vi "Self Fulfill Error.vi"(8 "error in (no error)":errorcluster) -> (0 "error out":errorcluster)   [LabVIEW 2017, in "Unit Tests.lvlib"]
uses:
  Unit Tests.lvlib
  e38c4525-3448-4fbc-8db8-7559fd649511.vi
  69632491-9656-44da-a05c-60cf6a618bb2.vi
  Promise Future/Promise/Promise.lvclass
  E:/Promise/Promise Future/Future/Future.lvclass
  Promise Future/Future/Fulfull (Future).vi
  Promise Future/Future/Read Value (private).vi
  <vilib>/addons/_JKI Toolkits/Caraya/classes/Test/Test.lvclass
  <vilib>/addons/_JKI Toolkits/Caraya/classes/Assert/Assert.lvclass
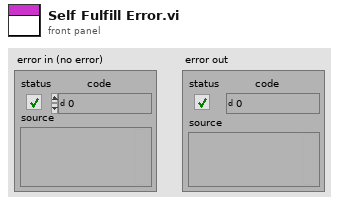
[diagram p1: front panel]
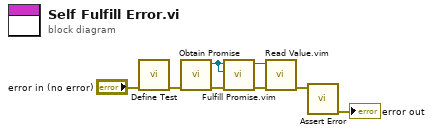
[diagram p0: block diagram]
diagram:
  n1 = call <vilib>:"Define Test.vi"("error in (no error)"="error in (no error)") -> ("error out"=w2:errorcluster)  [unwired: 10 in]
  n2 = call "Obtain Promise.vi"("error in (no error)"=w2) -> ("error out"=w5:errorcluster, "Promise out"=w6:refnum<class "Promise.lvclass">)  [unwired: 8 in, 1 out]
  n3 = call "Fulfill Promise.vim"("error in (no error)"=w5, "Value"=w6, "Promise in"=w6) -> ("error out"=w4:errorcluster, "Promise out"=w3:refnum<class "Promise.lvclass">)  [unwired: 7 in]
  n4 = call "Read Value.vim"("error in (no error)"=w4, "Future in"=w3) -> ("error out"=w1:errorcluster)  [unwired: 6 in, 3 out]
  n5 = call <vilib>:"Assert Error.vi"("Error?"=w1) -> ("error out"=→"error out":errorcluster)  [unwired: 10 in]
